vi "NicmosSetReadout.vi"(3 "READOUT in":T1, 9 "error in (no error)":errorcluster caption="error out (no error)") -> (0 "READOUT out":T1, 6 "error out":errorcluster)   [LabVIEW 2009]
uses:
  Controls/NICMOS.READOUT.ctl
  Controls/NICMOS.COMMAND.ctl
  Controls/NICMOS.COMMANDBASIC.ctl
  Controls/NICMOS.FILTERCOMMAND.ctl
  Controls/NICMOS.FILTER.ctl
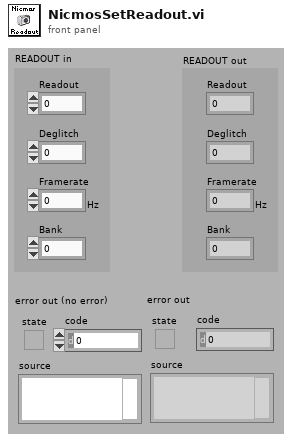
[diagram p1: front panel]
types:
  T1 = typedef "NICMOS.READOUT.ctl" = cluster{"Readout":i32, "Deglitch":i32, "Framerate":dbl[unit], "Bank":i32}
  T2 = typedef "NICMOS.COMMAND.ctl" = cluster{"Command":T3, "READOUT":T1, "FILTERCOMMAND":T4, "ACQUISITION":i32, "Done":refnum<k4>}
  T3 = typedef "NICMOS.COMMANDBASIC.ctl" = enum16{"WRITE BANKS", "SET FILTER", "HOME FILTER", "QUERY TEMP", "CONFIGURE", "START", "ACQUISITION", "STOP", "QUIT"}
  T4 = typedef "NICMOS.FILTERCOMMAND.ctl" = cluster{"FILTER":T5, "INIT":bool}
  T5 = typedef "NICMOS.FILTER.ctl" = string
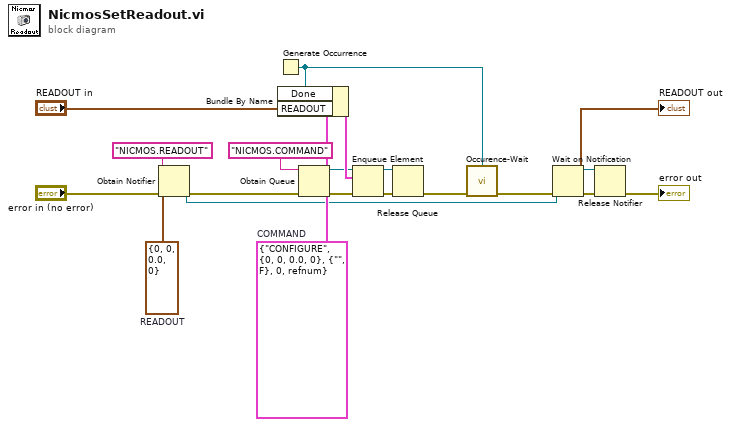
[diagram p0: block diagram]
diagram:
  w15 = T1 {"Readout"=0, "Deglitch"=0, "Framerate"=0.0, "Bank"=0}  # READOUT
  w17 = T2 {"Command"=enum."CONFIGURE", "READOUT"={"Readout"=0, "Deglitch"=0, "Framerate"=0.0, "Bank"=0}, "FILTERCOMMAND"={"FILTER"="", "INIT"=FALSE}, "ACQUISITION"=0, "Done"=refnum}  # COMMAND
  n1 = Obtain Notifier(name (unnamed)="NICMOS.READOUT" ("nom (aucun)"), notification data type=w15, error in (no error)="error in (no error)") -> (notifier out=w5:refnum<notifier>, error out=w2:errorcluster)  [unwired: 1 in, 1 out]
  n2 = Generate Occurrence() -> (w10:refnum<k4>)
  n3 = Bundle By Name(cluster=w17, "Done"=w10, "READOUT"="READOUT in") -> (w18:T2)
  n4 = Obtain Queue(name (unnamed)="NICMOS.COMMAND" ("nom (aucun)"), element data type=w17, error in (no error)=w2) -> (queue out=w9:refnum<queue>, error out=w7:errorcluster)  [unwired: 2 in, 1 out]
  n5 = Enqueue Element(queue=w9, element=w18, error in (no error)=w7) -> (queue out=w8:refnum<queue>, error out=w20:errorcluster)  [unwired: 1 in, 1 out]
  n6 = Release Queue(queue=w8, error in (no error)=w20) -> (error out=w13:errorcluster)  [unwired: 1 in, 2 out]
  n7 = call "Occurence-Wait.vi"("occurrence"=w10, "error out"=w13) -> ("error in (no error)"=w1:errorcluster)  [unwired: 7 in]
  n8 = Wait on Notification(notifier=w5, error in (no error)=w1) -> (notifier out=w4:refnum<notifier>, notification=→"READOUT out":T1, error out=w12:errorcluster)  [unwired: 2 in, 1 out]
  n9 = Release Notifier(notifier=w4, error in (no error)=w12) -> (error out=→"error out":errorcluster)  [unwired: 1 in, 2 out]
